vi "CurrentPath.vi"(8 "error in (no error)":errorcluster, 11 "Setting Database in":refnum<class "Setting Database.lvclass">) -> (0 "error out":errorcluster, 3 "Setting Database out":refnum<class "Setting Database.lvclass">)   [LabVIEW 2020, in "Setting Database.lvclass"]
uses:
  Setting Database.lvclass
  Path Settings/Path Settings.lvclass
panel:
  out "element":refnum<class "Path Settings.lvclass">
  in  "Index":i32
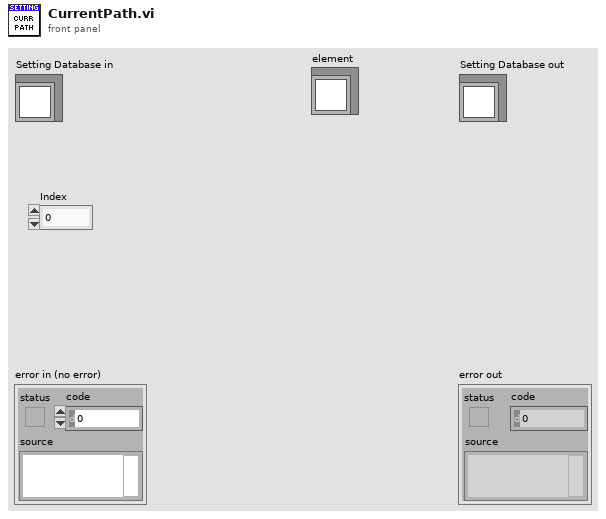
[diagram p1: front panel]
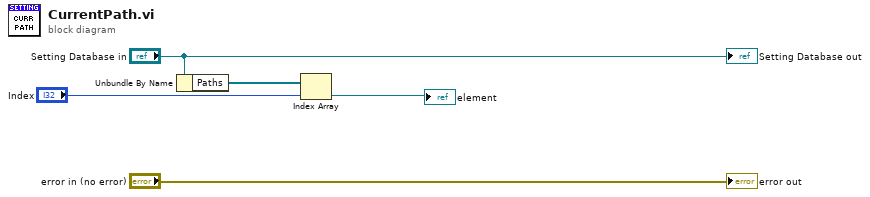
[diagram p0: block diagram]
diagram:
  n1 = Unbundle By Name("Setting Database in") -> ("Paths"=w4:refnum<class "Path Settings.lvclass">[])
  n2 = Index Array(array=w4, index="Index") -> (element=→"element":refnum<class "Path Settings.lvclass">)
  "error out" <- "error in (no error)"
  "Setting Database out" <- "Setting Database in"
